vi "GVmotor_get_move.vi"(8 "error in":errorcluster, 10 "wait_ms":u32=100, 11 "VISA in":refnum<visa-resource-name>) -> (0 "error out":errorcluster, 2 "Step":i32, 3 "VISA out":refnum<visa-resource-name>)   [LabVIEW 2019]
panel:
  out "i":i32
  out "raw string":string
  out "trimmed string":string
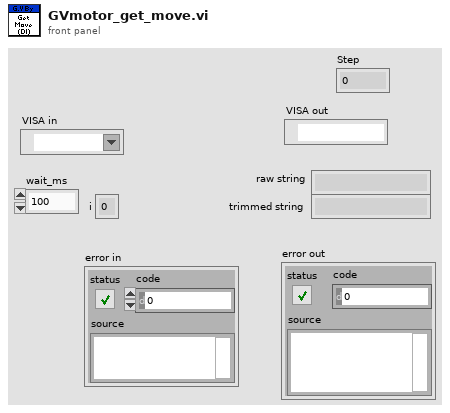
[diagram p1: front panel]
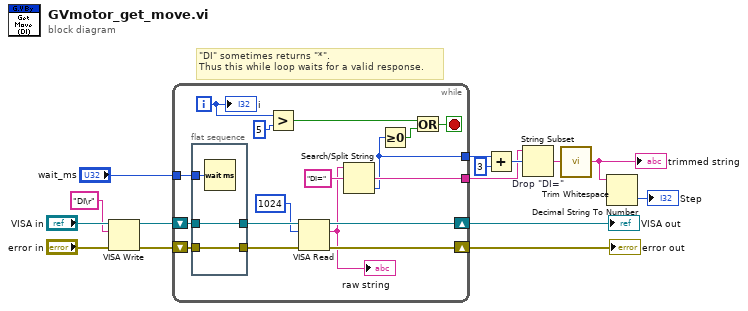
[diagram p0: block diagram]
diagram:
  # "\"DI\" sometimes returns \"*\".\nThus this while loop waits for a valid response."
  n1 = VISA Write(VISA resource name="VISA in", write buffer="DI\r" ("string"), error in (no error)="error in") -> (VISA resource name out=w12:refnum<visa-resource-name>, error out=w13:errorcluster)  [unwired: 1 out]
  n2 = while {
    tunnel: "wait_ms" -> [w28]
    shift-right: [w25] -> w7
    shift-left: w13 -> [w32]
    shift-right: [w27] -> w10
    shift-left: w12 -> [w31]
    tunnel: [w18] -> w4
    tunnel: [w16] -> w2
    i -> [w23]
    stop <- w21 stop-if-true
    n3 = flat-sequence {
      tunnel: [w35] -> w26
      tunnel: w32 -> [w35]
      tunnel: [w34] -> w30
      tunnel: w31 -> [w34]
      tunnel: w28 -> [w33]
      frame #0 {
        n4 = Wait (ms)(milliseconds to wait=w33) -> ()  [unwired: 1 out]
      }
    }
    n5 = Greater?(x=w23, y=5) -> (0:w20:bool)
    n6 = VISA Read(VISA resource name=w30, byte count=u32 1024, error in (no error)=w26) -> (VISA resource name out=w27:refnum<visa-resource-name>, read buffer=w19:string, error out=w25:errorcluster)  [unwired: 1 out]
    "raw string" <- w19
    n7 = Search/Split String(string=w19, search string/char (-)="DI=") -> (match + rest of string=w18:string, offset of match=w16:i32)  [unwired: 1 in, 1 out]
    n8 = Greater Or Equal To 0?(x=w16) -> (x >= 0?=w17:bool)
    n9 = Or(x=w20, y=w17) -> (x .or. y?=w21:bool)
    "i" <- w23
  }
  "error out" <- w7
  "VISA out" <- w10
  n10 = Add(x=w2, y=3) -> (x+y=w5:i32)
  n11 = String Subset "Drop \"DI=\""(string=w4, offset (0)=w5) -> (substring=w3:string)  [unwired: 1 in]
  n12 = call <vilib>:"Trim Whitespace.vi"("string"=w3) -> ("trimmed string"=w9:string)  [unwired: 1 in]
  "trimmed string" <- w9
  n13 = Decimal String To Number(string=w9) -> (number=→"Step":i32)  [unwired: 2 in, 1 out]
